vi "Main.vi"   [LabVIEW 2012]
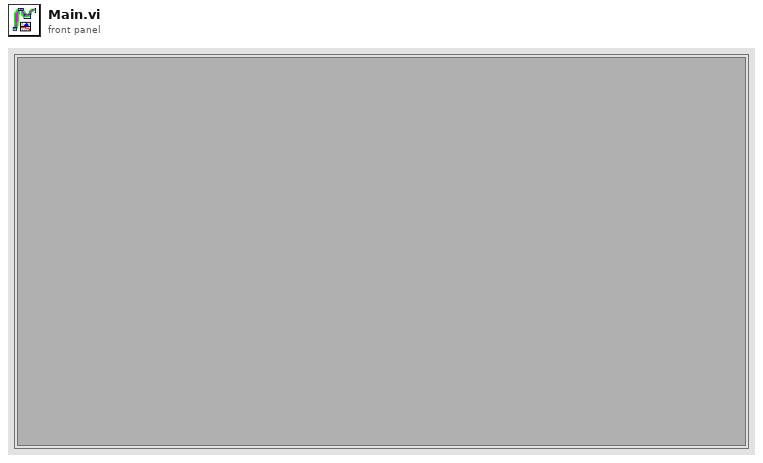
[diagram p1: front panel]
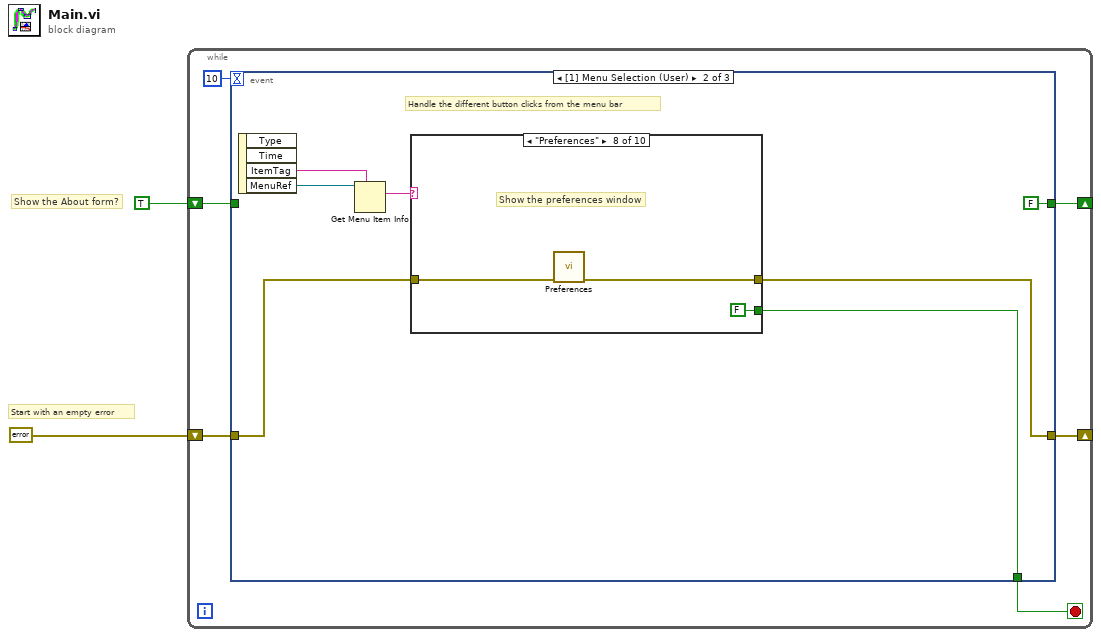
[diagram p0: block diagram]
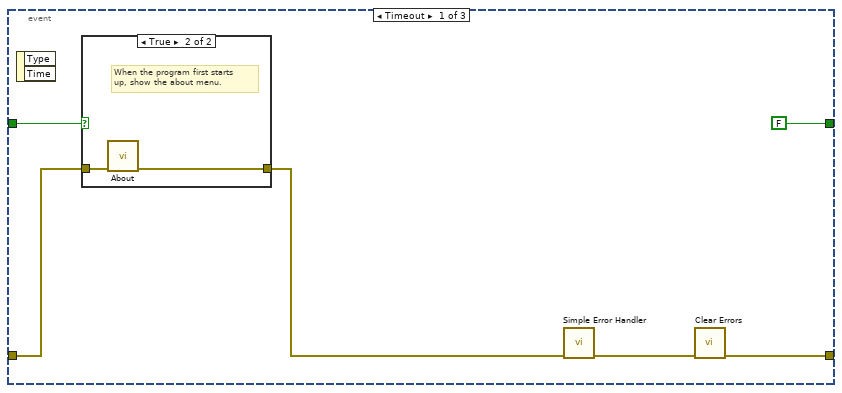
[diagram p2: hidden frame]
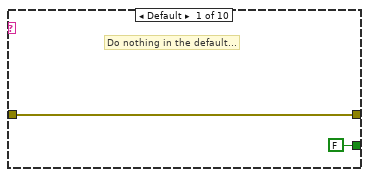
[diagram p4: hidden frame]
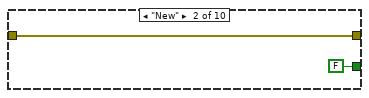
[diagram p5: hidden frame]
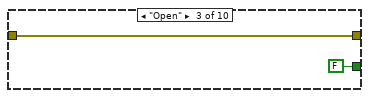
[diagram p6: hidden frame]
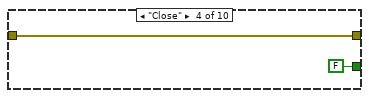
[diagram p7: hidden frame]
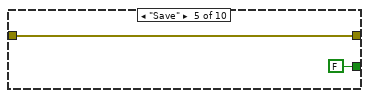
[diagram p8: hidden frame]
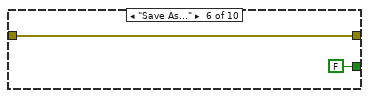
[diagram p9: hidden frame]
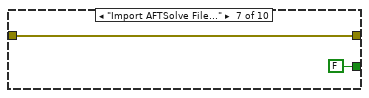
[diagram p10: hidden frame]
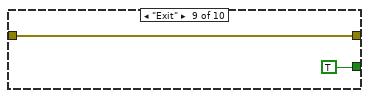
[diagram p11: hidden frame]
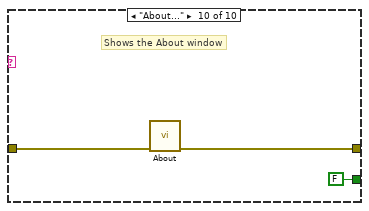
[diagram p12: hidden frame]
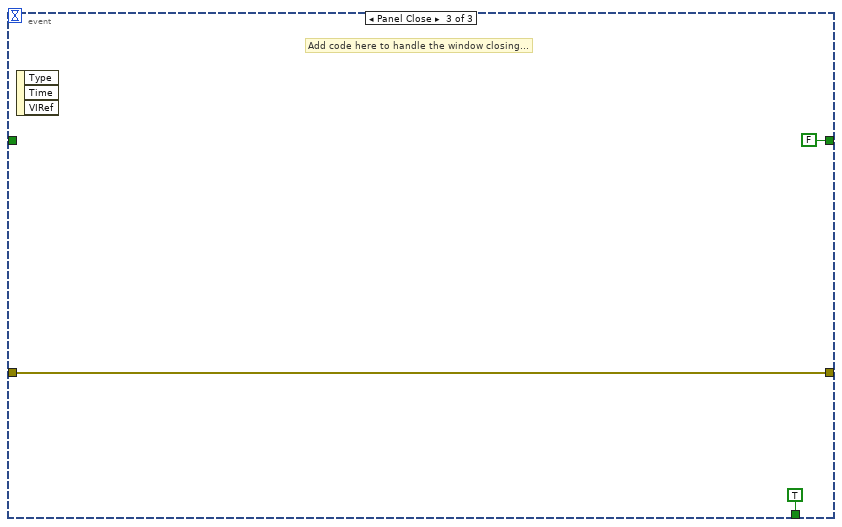
[diagram p13: hidden frame]
diagram:
  # "Start with an empty error"
  # "Show the About form?"
  n1 = while {
    shift-right: [w5] -> _
    shift-left: TRUE -> [w6]
    shift-right: [w3] -> _
    shift-left: errorcluster {"status"=FALSE, "code"=0, "source"=""} ("error constant") -> [w4]
    stop <- w8 stop-if-true
    n2 = event shown="[1] Menu Selection (User)" {
      selector: _ -> [_ _ _]
      dyn-events: _ -> [_ _ _]
      timeout: 10 -> [_ _ _]
      tunnel: [_ w21 TRUE] -> w8
      tunnel: w6 -> [w14 _ _]
      tunnel: [FALSE FALSE FALSE] -> w5
      tunnel: w4 -> [w10 w20 w48]
      tunnel: [w11 w19 w48] -> w3
      event Timeout {
        n3 = event-data() -> ()  [unwired: 1 in, 2 out]
        n4 = case shown="True" w14 {
          tunnel: w10 -> [w15 w17]
          tunnel: [w15 w16] -> w9
          frame False {
          }
          frame True {
            # "When the program first starts\nup, show the about menu."
            n5 = call "About.vi"("error in (no error)"=w17) -> ("error out"=w16:errorcluster)  [unwired: 10 in]
          }
        }
        n6 = call <vilib>:"Simple Error Handler.vi"("error in (no error)"=w9) -> ("error out"=w12:errorcluster)  [unwired: 4 in, 4 out]
        n7 = call <vilib>:"Clear Errors.vi"("error in (no error)"=w12) -> ("error out"=w11:errorcluster)  [unwired: 6 in]
      }
      event Menu Selection (User) {
        # "Handle the different button clicks from the menu bar"
        n8 = event-data() -> ("ItemTag"=w23:string, "MenuRef"=w24:refnum<k9>)  [unwired: 1 in, 2 out]
        n9 = Get Menu Item Info(7:w23, 11:w24) -> (2:w22:string)  [unwired: 1 in, 6 out]
        n10 = case shown="\"Preferences\"" w22 {
          tunnel: [FALSE FALSE FALSE FALSE FALSE FALSE FALSE FALSE TRUE FALSE] -> w21
          tunnel: w20 -> [w25 w27 w29 w31 w33 w35 w37 w40 w42 w45]
          tunnel: [w25 w27 w29 w31 w33 w35 w37 w39 w42 w44] -> w19
          frame Default {
            # "Do nothing in the default..."
          }
          frame "New" {
          }
          frame "Open" {
          }
          frame "Close" {
          }
          frame "Save" {
          }
          frame "Save As..." {
          }
          frame "Import AFTSolve File..." {
          }
          frame "Preferences" {
            # "Show the preferences window"
            n11 = call "Preferences.vi"("error in (no error)"=w40) -> ("error out"=w39:errorcluster)  [unwired: 10 in]
          }
          frame "Exit" {
          }
          frame "About..." {
            # "Shows the About window"
            n12 = call "About.vi"("error in (no error)"=w45) -> ("error out"=w44:errorcluster)  [unwired: 10 in]
          }
        }
      }
      event Panel Close {
        # "Add code here to handle the window closing..."
        n13 = event-data() -> ()  [unwired: 1 in, 3 out]
      }
    }
  }
